vi "Timestamp to Unix Epoch.vi"(10 "error in (no error)":errorcluster, 11 "Time Stamp":timestamp) -> (2 "error out":errorcluster, 3 "Unix Epoch Seconds":dbl format="%#.6f")   [LabVIEW 2020, in "JWT.lvlib"]
uses:
  JWT.lvlib
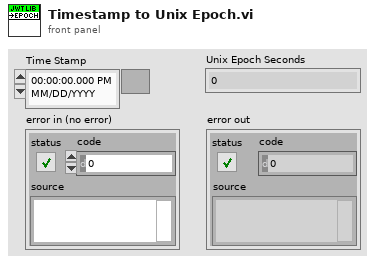
[diagram p1: front panel]
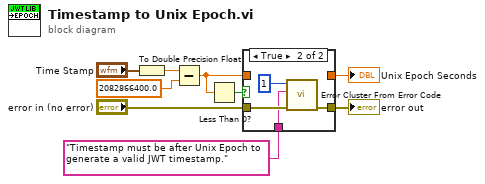
[diagram p0: block diagram]
diagram:
  n1 = To Double Precision Float(number="Time Stamp") -> (double precision float=w8:dbl)
  n2 = Subtract(x=w8, y=2082866400.0 ("double precision float")) -> (x-y=w5:dbl)
  n3 = Less Than 0?(x=w5) -> (x < 0?=w6:bool)
  n4 = case shown="True" w6 {
    tunnel: w5 -> [w10 _]
    tunnel: [w10 _] -> w4
    tunnel: "error in (no error)" -> [w11 w15]
    tunnel: [w11 w13] -> w2
    tunnel: "Timestamp must be after Unix Epoch to generate a valid JWT timestamp." -> [_ w12]
    frame False {
    }
    frame True {
      n5 = call <vilib>:"Error Cluster From Error Code.vi"("error in (no error)"=w15, "error message (\"\")"=w12, "error code (0)"=1) -> ("error out"=w13:errorcluster)  [unwired: 6 in]
    }
  }
  "Unix Epoch Seconds" <- w4
  "error out" <- w2
